vi "DqmhModuleDiagramGraph_GetObjectStatus.vi"(0 "reference in":refnum<class "DqmhModuleDiagramGraph.lvclass">, 5 "error in (no error)":errorcluster) -> (10 "# of objects":i32, 11 "Not a refnum?":bool, 12 "All objects names":string[](array[string]), 13 "Class name":string, 14 "reference out":refnum<class "DqmhModuleDiagramGraph.lvclass">, 15 "Object name":string, 16 "All refs out":refnum<class "DqmhModuleDiagramGraph.lvclass">[](array[class]), 19 "error out":errorcluster)   [LabVIEW 2014, in "DqmhModuleDiagramGraph.lvclass"]
doc: "Returns the object status and also information about all the objects in the class."
uses:
  <resource>/Framework/Providers/Open_GDS/UML/DqmhModuleDiagramGraph_class/DqmhModuleDiagramGraph.lvclass
  <resource>/Framework/Providers/Open_GDS/UML/DqmhModuleDiagramGraph_class/protected/ObjectAttributes.ctl
  <resource>/Framework/Providers/Open_GDS/UML/DqmhModuleDiagramGraph_class/protected/ClassAttributes.ctl
  <resource>/Framework/Providers/Open_GDS/UML/Graph_class/protected/ClassAttributes.ctl
  <resource>/Framework/Providers/Open_GDS/UML/AbstractNode_class/AbstractNode.lvclass
  <resource>/Framework/Providers/Open_GDS/UML/AbstractEdge_class/AbstractEdge.lvclass
  <resource>/Framework/Providers/Open_GDS/UML/Graph_class/Graph.lvclass
panel:
  in  "DebuggerInput":variant
  out "DebuggerOutput":variant
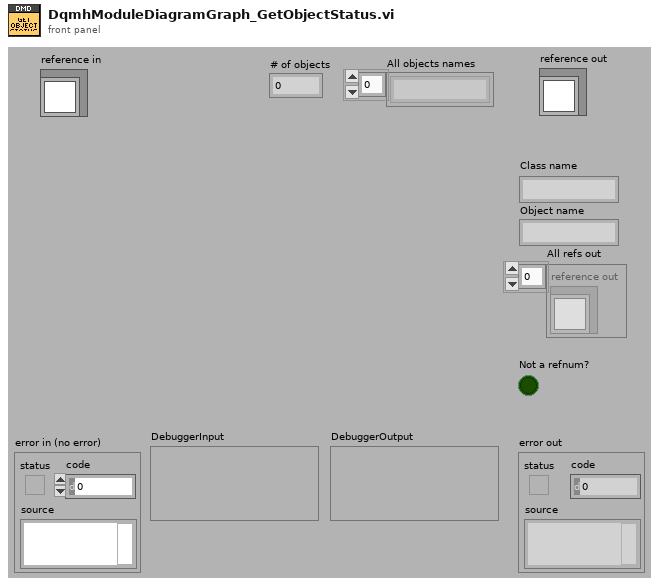
[diagram p1: front panel]
types:
  T1 = typedef "DqmhModuleDiagramGraph.lvclass/ClassAttributes.ctl" = cluster{"Base class":T2}
  T2 = typedef "Graph.lvclass/ClassAttributes.ctl" = cluster{"NODE_PROT":refnum<class "AbstractNode.lvclass">[], "NodeNames":string[], "EDGE_PROT":refnum<class "AbstractEdge.lvclass">[], "EdgeNames":string[], "GraphTypes":refnum<class "Graph.lvclass">[], "GraphTypeNames":string[], "NodeTypes":refnum<class "AbstractNode.lvclass">[], "EdgeTypes":refnum<class "AbstractEdge.lvclass">[], "NodeTypeNames":string[], "EdgeTypeNames":string[]}
  T3 = typedef "DqmhModuleDiagramGraph.lvclass/ObjectAttributes.ctl" = cluster{"None":bool}
  T4 = cluster{"Mode":enum16{"Get", "Set", "Delete"}, "Ref":variant, "ObjAttribute":string, "ClassAttribute":string}
  T5 = cluster{"Object names":string[], "Refs":variant, "ObjectAttributeLocked":bool, "ClassAttributeLocked":bool, "ObjAttribute":variant, "ClassAttribute":variant}
  T6 = typedef "ClassDiagramGraph.lvclass/ObjectAttributes.ctl" = cluster{"None":bool}
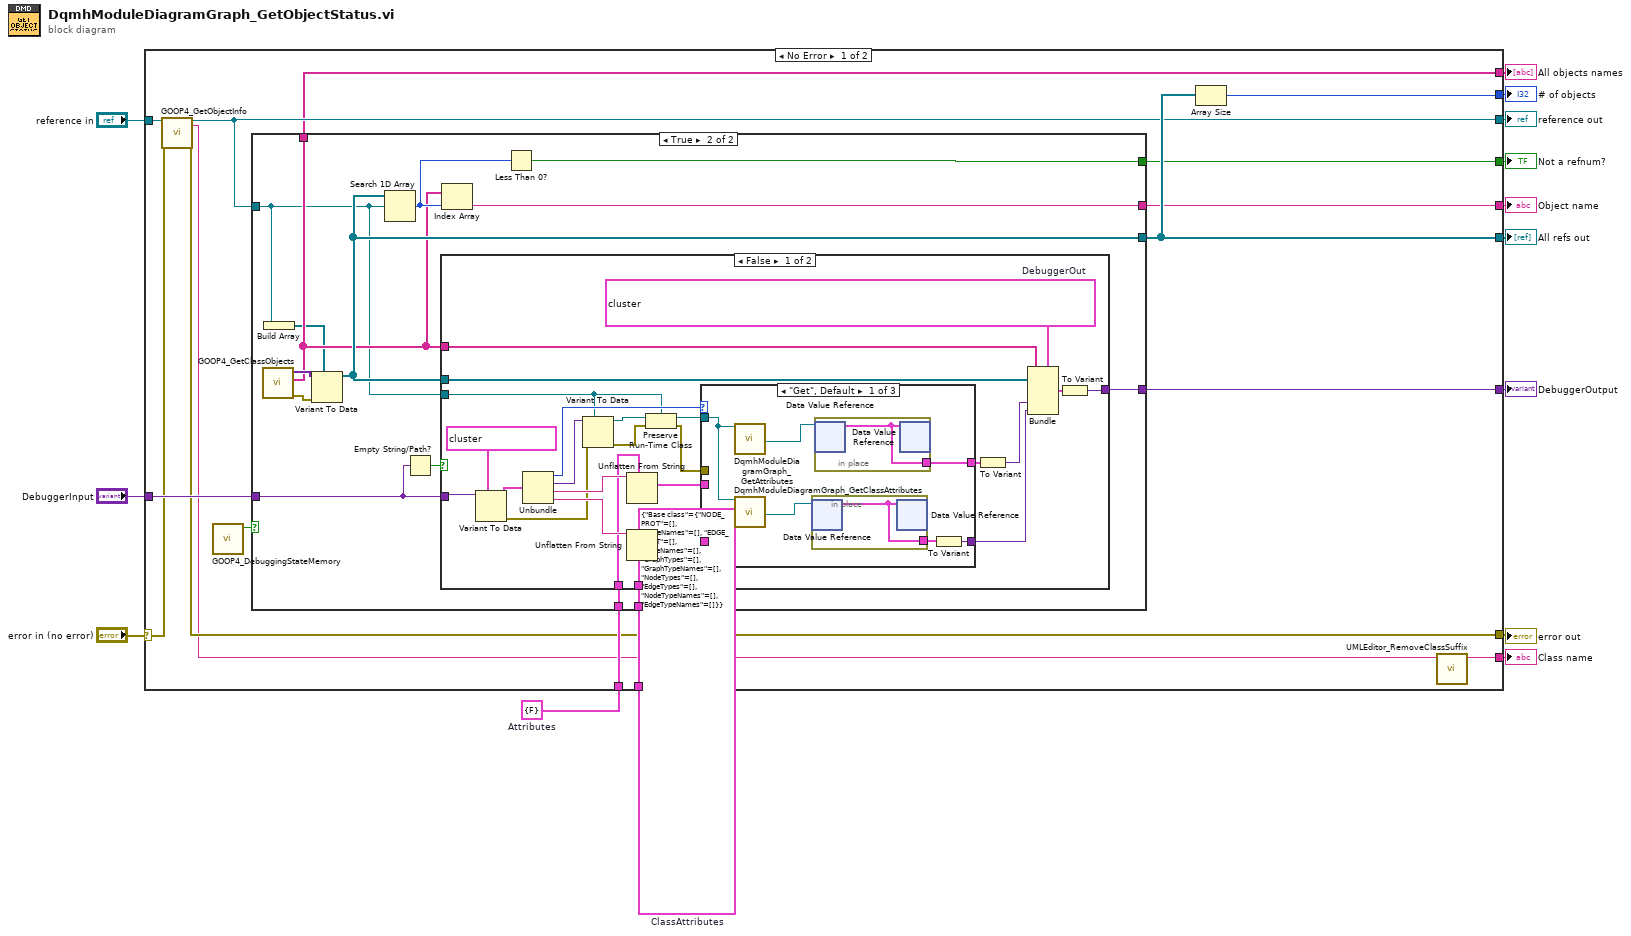
[diagram p0: block diagram]
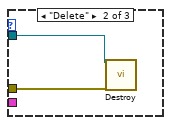
[diagram p3: hidden frame]
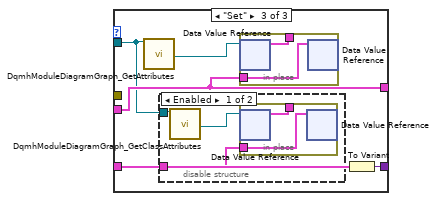
[diagram p4: hidden frame]
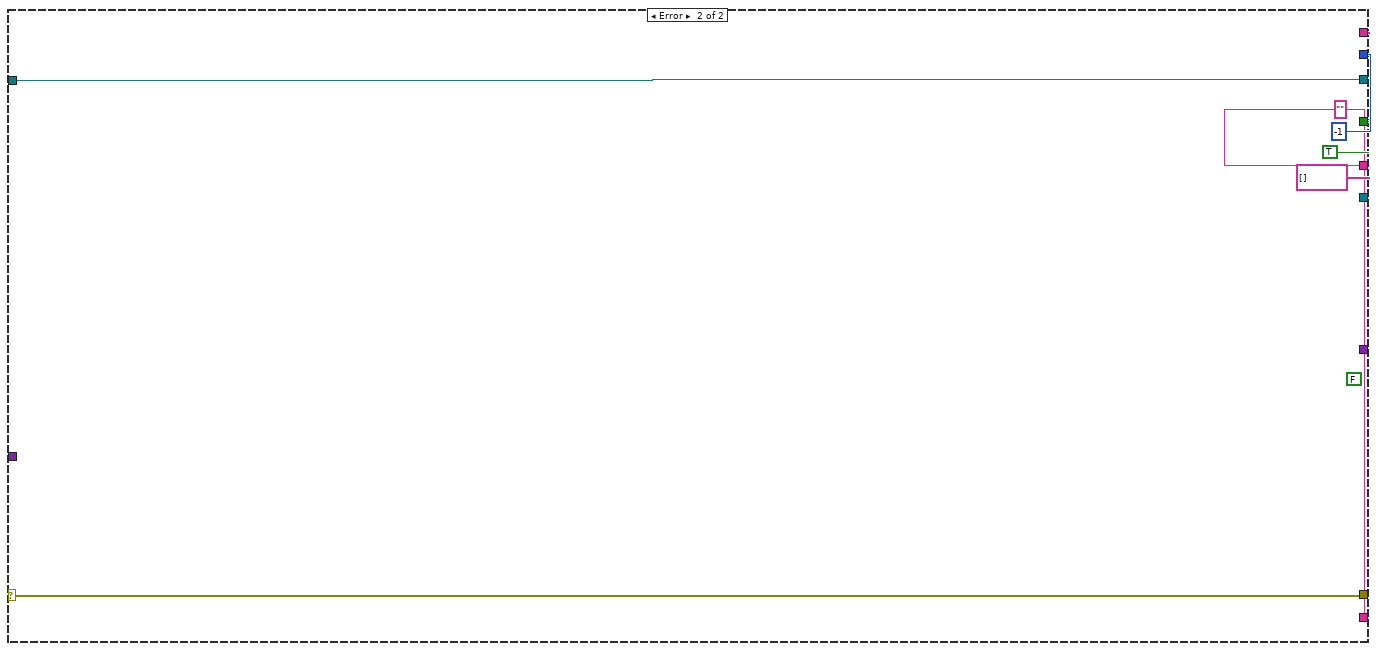
[diagram p7: hidden frame]
diagram:
  w2 = T1 {"Base class"={"NODE_PROT"=[], "NodeNames"=[], "EDGE_PROT"=[], "EdgeNames"=[], "GraphTypes"=[], "GraphTypeNames"=[], "NodeTypes"=[], "EdgeTypes"=[], "NodeTypeNames"=[], "EdgeTypeNames"=[]}}  # ClassAttributes
  w3 = T3 {"None"=FALSE}  # Attributes
  n1 = case shown="No Error" "error in (no error)" {
    selector: "error in (no error)" -> [w26 w92]
    tunnel: "reference in" -> [w28 w96]
    tunnel: [w21 w96] -> w12
    tunnel: [w30 -1 ("# of objects")] -> w1
    tunnel: [w19 TRUE ("Exists?")] -> w11
    tunnel: [w15 w93] -> w10
    tunnel: [w17 string[] [] ("Object names")] -> w9
    tunnel: [w20 w93] -> w8
    tunnel: "DebuggerInput" -> [w27 _]
    tunnel: [w29 _] -> w6
    tunnel: [w23 _] -> w5
    tunnel: w3 -> [w25 _]
    tunnel: w2 -> [w24 _]
    tunnel: [w18 w92] -> w4
    frame No Error {
      n2 = call <vilib>:"GOOP4_GetObjectInfo.vi"("ObjectIn"=w28, "error in (no error)"=w26) -> ("ObjectOut"=w21:refnum<class "DqmhModuleDiagramGraph.lvclass">, "ObjectRuntimeClassName"=w16:string, "error out"=w18:errorcluster)  [unwired: 12 in, 3 out]
      n3 = call <vilib>:"GOOP4_DebuggingStateMemory.vi"() -> ("CurrentDebuggingState"=w22:bool)  [unwired: 10 in, 1 out]
      n4 = case shown="True" w22 {
        tunnel: w27 -> [_ w43]
        tunnel: [_ w42] -> w29
        tunnel: w25 -> [_ w41]
        tunnel: w24 -> [_ w40]
        tunnel: [_ w35] -> w23
        tunnel: [_ w33] -> w17
        tunnel: w21 -> [_ w32]
        tunnel: [_ w37] -> w20
        tunnel: [_ w36] -> w19
        frame False {
        }
        frame True {
          n5 = call <vilib>:"GOOP4_GetClassObjects.vi"() -> ("error out"=w38:errorcluster, "ObjectNames"=w33:string[], "ObjectsRefs"=w39:variant[])  [unwired: 9 in]
          n6 = Build Array(w32) -> (w31:refnum<class "DqmhModuleDiagramGraph.lvclass">[])
          n7 = Variant To Data(error in=w38, type=w31, Variant=w39) -> (data=w35:refnum<class "DqmhModuleDiagramGraph.lvclass">[])  [unwired: 1 out]
          n8 = Search 1D Array(1D array=w35, element=w32) -> (index of element=w34:i32)  [unwired: 1 in]
          n9 = Empty String/Path?(string/path=w43) -> (empty?=w44:bool)
          n10 = case shown="False" w44 {
            tunnel: [w46 _] -> w42
            tunnel: w41 -> [w66 _]
            tunnel: w40 -> [w65 _]
            tunnel: w43 -> [w58 _]
            tunnel: w35 -> [w54 _]
            tunnel: w33 -> [w60 _]
            tunnel: w32 -> [w53 _]
            frame False {
              w59 = T5 {"Object names"=[], "Refs"=variant, "ObjectAttributeLocked"=FALSE, "ClassAttributeLocked"=FALSE, "ObjAttribute"=variant, "ClassAttribute"=variant}  # DebuggerOut
              n11 = Variant To Data(type=T4 {"Mode"=enum."Delete", "Ref"=variant, "ObjAttribute"="", "ClassAttribute"=""} ("DebuggerIn"), Variant=w58) -> (data=w56:T4, error out=w48:errorcluster)  [unwired: 1 in]
              n12 = Unbundle(w56) -> ("Mode"=w64:enum16{"Get", "Set", "Delete"}, "Ref"=w55:variant, "ObjAttribute"=w68:string, "ClassAttribute"=w69:string)
              n13 = Variant To Data(error in=w48, type=w53, Variant=w55) -> (data=w52:refnum<class "DqmhModuleDiagramGraph.lvclass">, error out=w50:errorcluster)
              n14 = Unflatten From String(type=w66, binary string=w68) -> (value=w67:T3)  [unwired: 3 in, 2 out]
              n15 = Unflatten From String(type=w65, binary string=w69) -> (value=w63:T1)  [unwired: 3 in, 2 out]
              n16 = Preserve Run-Time Class(object in=w52, error in=w50, 2:w53) -> (object out=w51:refnum<class "DqmhModuleDiagramGraph.lvclass">, error out=w49:errorcluster)
              n17 = case shown="\"Get\", Default" w64 {
                tunnel: w51 -> [w73 w79 w80]
                tunnel: [w75 _ w83] -> w61
                tunnel: [w70 _ w82] -> w45
                tunnel: w67 -> [_ _ w83]
                tunnel: w63 -> [_ _ w81]
                tunnel: w49 -> [_ w78 _]
                frame "Get", Default {
                  n18 = call <resource>:"DqmhModuleDiagramGraph_GetAttributes.vi"("reference in"=w73) -> ("DataRef"=w74:refnum<data-value>)  [unwired: 15 in, 3 out]
                  n19 = call <resource>:"DqmhModuleDiagramGraph_GetClassAttributes.vi"("reference in"=w73) -> ("Class attribute Reference"=w72:refnum<data-value>)  [unwired: 15 in, 3 out]
                  n20 = in-place {
                    in-place-border: [w76] -> w71
                    n21 = in-place-dvr #1(w72) -> (w76:T1)  [unwired: 1 out]
                    n22 = in-place-dvr #1(w76) -> ()  [unwired: 2 out]
                  }
                  n23 = in-place {
                    in-place-border: [w77] -> w75
                    n24 = in-place-dvr #2(w74) -> (w77:T6)  [unwired: 1 out]
                    n25 = in-place-dvr #2(w77) -> ()  [unwired: 2 out]
                  }
                  n26 = To Variant(anything=w71) -> (Variant=w70:variant)
                }
                frame "Delete" {
                  n27 = call-dynamic "Destroy.vi"("reference in"=w79, "error in (no error)"=w78) -> ()  [unwired: 17 in, 1 out]
                }
                frame "Set" {
                  n28 = call <resource>:"DqmhModuleDiagramGraph_GetAttributes.vi"("reference in"=w80) -> ("DataRef"=w84:refnum<data-value>)  [unwired: 15 in, 3 out]
                  n29 = disable-structure shown="Enabled" {
                    disable-tunnel: w81 -> [w86 _]
                    disable-tunnel: w80 -> [w85 _]
                    frame Enabled {
                      n30 = call <resource>:"DqmhModuleDiagramGraph_GetClassAttributes.vi"("reference in"=w85) -> ("Class attribute Reference"=w87:refnum<data-value>)  [unwired: 15 in, 3 out]
                      n31 = in-place {
                        in-place-border: w86 -> [w89]
                        in-place-border: [w88] -> _
                        n32 = in-place-dvr #3(w87) -> (w88:T1)  [unwired: 1 out]
                        n33 = in-place-dvr #3(w89) -> ()  [unwired: 2 out]
                      }
                    }
                    frame Disabled {
                    }
                  }
                  n34 = in-place {
                    in-place-border: w83 -> [w91]
                    in-place-border: [w90] -> _
                    n35 = in-place-dvr #4(w84) -> (w90:T6)  [unwired: 1 out]
                    n36 = in-place-dvr #4(w91) -> ()  [unwired: 2 out]
                  }
                  n37 = To Variant(anything=w81) -> (Variant=w82:variant)
                }
              }
              n38 = To Variant(anything=w61) -> (Variant=w62:variant)
              n39 = Bundle(cluster=w59, "Object names"=w60, "Refs"=w54, "ObjAttribute"=w62, "ClassAttribute"=w45) -> (w47:T5)  [unwired: 2 in]
              n40 = To Variant(anything=w47) -> (Variant=w46:variant)
            }
            frame True {
            }
          }
          n41 = Index Array(array=w33, index=w34) -> (element=w37:string)
          n42 = Less Than 0?(x=w34) -> (x < 0?=w36:bool)
        }
      }
      n43 = Array Size(array=w23) -> (size(s)=w30:i32)
      n44 = call <resource>:"UMLEditor_RemoveClassSuffix.vi"("ObjectRuntimeClassName in"=w16) -> ("ObjectRuntimeClassName out"=w15:string)  [unwired: 10 in]
    }
    frame Error {
      w93 = "" ("Class name")
      (unwired) FALSE
    }
  }
  "error out" <- w4
  "reference out" <- w12
  "# of objects" <- w1
  "Not a refnum?" <- w11
  "All refs out" <- w5
  "Class name" <- w10
  "All objects names" <- w9
  "Object name" <- w8
  "DebuggerOutput" <- w6
